vi "SubVI_ConversõesPraMetro.vi"(4 "error in":errorcluster, 5 "km":dbl format="%#_13g", 6 "cm":dbl format="%#_13g", 7 "mm":dbl format="%#_13g") -> (0 "error out":errorcluster, 1 "km para metros":dbl, 2 "cm para metros":dbl, 3 "mm para metros":dbl)   [LabVIEW 2023]
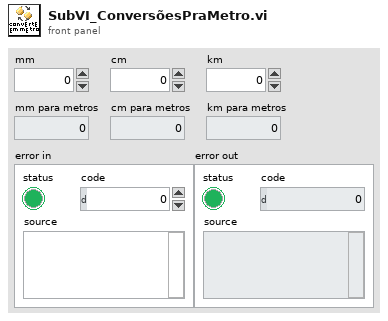
[diagram p1: front panel]
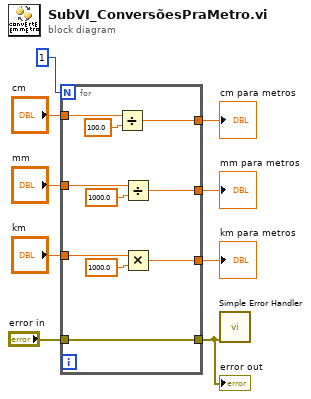
[diagram p0: block diagram]
diagram:
  n1 = for {
    N: 1 -> [_]
    tunnel: [w19] -> w8
    tunnel: "error in" -> [w19]
    tunnel: "km" -> [w15]
    tunnel: "cm" -> [w14]
    tunnel: "mm" -> [w13]
    tunnel: [w12] -> w3
    tunnel: [w11] -> w2
    tunnel: [w10] -> w1
    n2 = Divide(x=w14, y=100.0) -> (x/y=w11:dbl)
    n3 = Divide(x=w13, y=1000.0) -> (x/y=w12:dbl)
    n4 = Multiply(x=w15, y=1000.0) -> (x*y=w10:dbl)
  }
  "error out" <- w8
  "mm para metros" <- w3
  "cm para metros" <- w2
  "km para metros" <- w1
  n5 = call <vilib>:"Simple Error Handler.vi"("error in (no error)"=w8) -> ()  [unwired: 4 in, 5 out]
